vi "Simple UDP Server.vi"() -> ()   [LabVIEW 2014, in "ESP8266 WiFi Wrapper.lvlib"]
uses:
  ESP8266 WiFi Wrapper.lvlib
  <vilib>/Aledyne-TSXperts/Arduino Compatible Compiler for LabVIEW/Arduino Compatible Compiler for LabVIEW.lvlib
panel:
  in  "DNS address":u8[](array[numeric])=[0, 0, 0, 0]
  in  "IP address":u8[](array[numeric])=[192, 168, 0, 47]
  in  "Gateway":u8[](array[numeric])=[192, 168, 0, 1]
  in  "Subnet mask":u8[](array[numeric])=[255, 255, 255, 0]
  in  "Password":string="12345678"
  in  "SSID":string="ESP8266 Wifi UDP"
  in  "Listen Port":i16=8080
  in  "error in (no error)":errorcluster
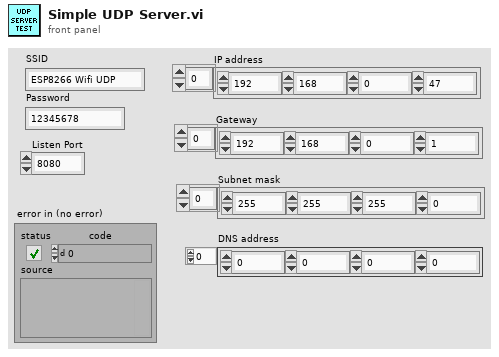
[diagram p1: front panel]
types:
  T1 = enum8{"WIFI_OFF", "WIFI_STA", "WIFI_AP", "WIFI_AP_STA"}
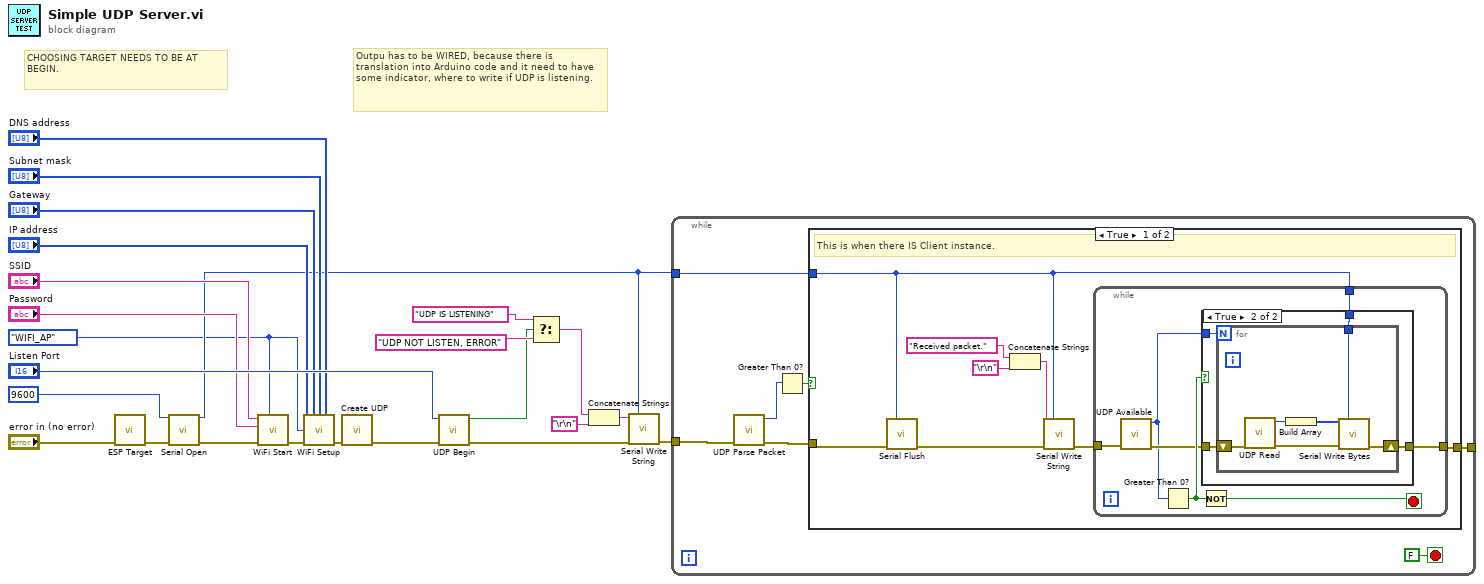
[diagram p0: block diagram]
diagram:
  w1 = T1."WIFI_AP" ("Enum")
  # "Outpu has to be WIRED, because there is translation into Arduino code and it need to have some indicator, where to write if UDP is listening."
  # "CHOOSING TARGET NEEDS TO BE AT BEGIN."
  n1 = call "ESP Target.vi"("Error In"="error in (no error)") -> ("Error Out"=w23:errorcluster)  [unwired: 10 in]
  n2 = call <vilib>:"Serial Open.vi"("Speed"=u32 9600, "error in (no error)"=w23) -> ("Instance"=w8:u8, "error out"=w13:errorcluster)  [unwired: 12 in]
  n3 = call "WiFi Start.vi"("WiFi Mode"=w1, "Error In"=w13, "Password"="Password", "SSID"="SSID") -> ("Error Out"=w12:errorcluster)  [unwired: 7 in]
  n4 = call "WiFi Setup.vi"("IP address"="IP address", "Gateway address"="Gateway", "Subnet mask"="Subnet mask", "DNS address"="DNS address", "WiFi Mode"=w1, "Error In"=w12) -> ("Error Out"=w16:errorcluster)  [unwired: 9 in]
  n5 = call "Create UDP.vi"("Error In"=w16) -> ("Error Out"=w11:errorcluster)  [unwired: 10 in]
  n6 = call "UDP Begin.vi"("Error In"=w11, "Port"="Listen Port") -> ("Error Out"=w9:errorcluster, "Is listening?"=w5:bool)  [unwired: 8 in]
  n7 = Select(t="UDP IS LISTENING", s=w5, f="UDP NOT LISTEN, ERROR") -> (s? t:f=w2:string)
  n8 = Concatenate Strings(w2, "\r\n") -> (w4:string)
  n9 = call <vilib>:"Serial Write String.vi"("String"=w4, "Instance"=w8, "error in (no error)"=w9) -> ("error out"=w10:errorcluster)  [unwired: 12 in]
  n10 = while {
    tunnel: w10 -> [w26]
    tunnel: w8 -> [w30]
    tunnel: [w25] -> _
    stop <- FALSE stop-if-true
    n11 = call "UDP Parse Packet.vi"("Error In"=w26) -> ("Error Out"=w27:errorcluster, "Size of packet in bytes"=w28:i32)  [unwired: 9 in]
    n12 = Greater Than 0?(x=w28) -> (x > 0?=w29:bool)
    n13 = case shown="True" w29 {
      tunnel: w30 -> [w32 _]
      tunnel: w27 -> [w38 w58]
      tunnel: [w33 w58] -> w25
      frame True {
        # "This is when there IS Client instance."
        n14 = call <vilib>:"Serial Flush.vi"("Instance"=w32, "error in (no error)"=w38) -> ("error out"=w39:errorcluster)  [unwired: 13 in]
        n15 = Concatenate Strings("Received packet." ("String"), "\r\n") -> (w36:string)
        n16 = call <vilib>:"Serial Write String.vi"("String"=w36, "Instance"=w32, "error in (no error)"=w39) -> ("error out"=w34:errorcluster)  [unwired: 12 in]
        n17 = while {
          tunnel: w34 -> [w46]
          tunnel: [w43] -> w33
          tunnel: w32 -> [w41]
          stop <- w45 stop-if-true
          n18 = call "UDP Available.vi"("Error In"=w46) -> ("Error Out"=w42:errorcluster, "Available?"=w40:u8)  [unwired: 9 in]
          n19 = Greater Than 0?(x=w40) -> (x > 0?=w44:bool)
          n20 = Not(x=w44) -> (.not. x?=w45:bool)
          n21 = case shown="True" w44 {
            tunnel: [w47 w50] -> w43
            tunnel: w42 -> [w47 w51]
            tunnel: w41 -> [_ w49]
            tunnel: w40 -> [_ w48]
            frame False {
            }
            frame True {
              n22 = for {
                N: w48 -> [_]
                tunnel: w49 -> [w52]
                shift-right: [w55] -> w50
                shift-left: w51 -> [w57]
                n23 = call "UDP Read.vi"("Error In"=w57) -> ("Error Out"=w56:errorcluster, "Read byte"=w54:u8)  [unwired: 9 in]
                n24 = Build Array(w54) -> (w53:u8[])
                n25 = call <vilib>:"Serial Write Bytes.vi"("Data"=w53, "Instance"=w52, "error in (no error)"=w56) -> ("error out"=w55:errorcluster)  [unwired: 12 in]
              }
            }
          }
        }
      }
      frame False {
        # "No Client instance, do nothing."
      }
    }
  }
